vi "get_instances.vi"(6 "id (unnamed)":string, 8 "error in (no error)":errorcluster, 10 "Base Class (LabVIEW Object)":refnum<class>, 11 "Mapped Lookup in":refnum<class "Mapped Lookup.lvclass">) -> (0 "error out":errorcluster, 2 "instances":set{refnum<data-value>}(c389), 3 "Mapped Lookup out":refnum<class "Mapped Lookup.lvclass">)   [LabVIEW 2019, in "LVCOOOP.lvlib" / "Lookup API.lvlib" / "Mapped Lookup.lvclass"]
uses:
  Mapped Lookup.lvclass
  Mapped Lookup.lvclass/Mapped Lookup.ctl
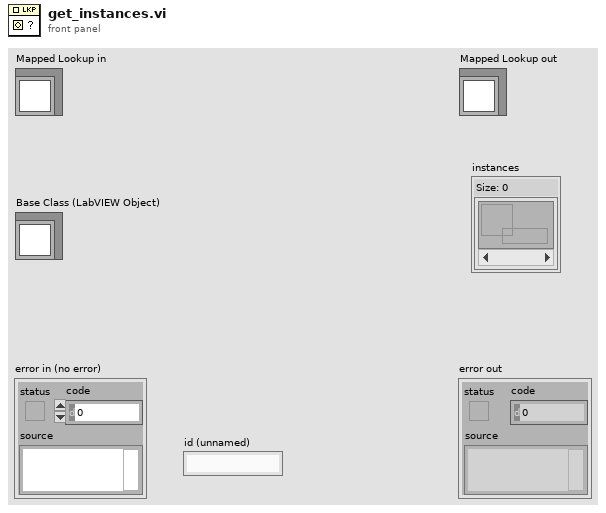
[diagram p1: front panel]
types:
  T1 = map{string, cluster{"instances":refnum<data-value>, "events":refnum<data-value>}}
  T2 = cluster{"instances":refnum<data-value>, "events":refnum<data-value>}
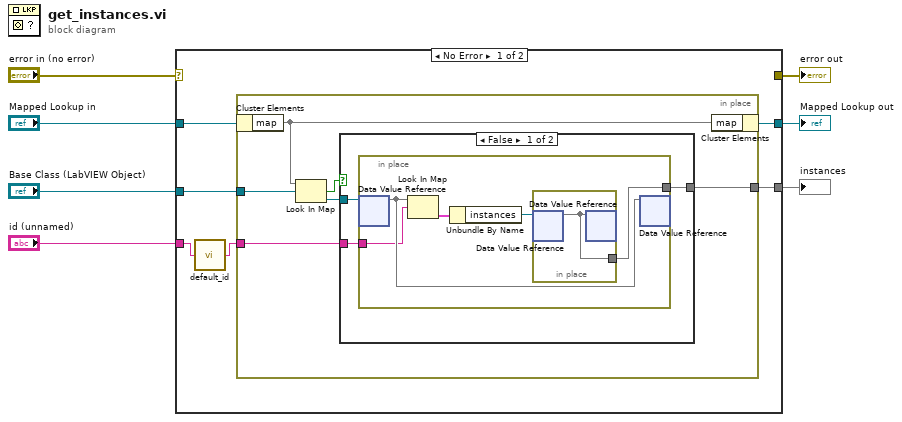
[diagram p0: block diagram]
diagram:
  n1 = case shown="No Error" "error in (no error)" {
    selector: "error in (no error)" -> [_ w30]
    tunnel: [_ w30] -> w6
    tunnel: [w10 w29] -> w5
    tunnel: "Mapped Lookup in" -> [w12 w29]
    tunnel: "id (unnamed)" -> [w13 _]
    tunnel: "Base Class (LabVIEW Object)" -> [w11 _]
    tunnel: [w8 _] -> w1
    frame No Error {
      n2 = call "default_id.vi"("id (unnamed)"=w13) -> ("String"=w9:string)
      n3 = in-place {
        in-place-border: w11 -> [w19]
        in-place-border: w9 -> [w15]
        in-place-border: [w14] -> w8
        n4 = in-place-cluster #1(w12) -> ("map"=w17:map{refnum<class>, refnum<data-value>})
        n5 = Look In Map(map=w17, key=w19) -> (key not found?=w18:bool, value=w16:refnum<data-value>)  [unwired: 1 in]
        n6 = case shown="False" w18 {
          tunnel: w16 -> [w22 _]
          tunnel: w15 -> [w21 _]
          tunnel: [w20 _] -> w14
          frame False {
            n7 = in-place {
              in-place-border: w21 -> [w26]
              in-place-border: [w23] -> w20
              n8 = in-place-dvr #2(w22) -> (w27:T1)  [unwired: 1 out]
              n9 = Look In Map(map=w27, key=w26) -> (value=w25:T2)  [unwired: 1 in, 1 out]
              n10 = Unbundle By Name(w25) -> ("instances"=w24:refnum<data-value>)
              n11 = in-place {
                in-place-border: [w28] -> w23
                n12 = in-place-dvr #3(w24) -> (w28:set{refnum<data-value>})  [unwired: 1 out]
                n13 = in-place-dvr #3(w28) -> ()  [unwired: 2 out]
              }
              n14 = in-place-dvr #2(w27) -> ()  [unwired: 2 out]
            }
          }
          frame True {
          }
        }
        n15 = in-place-cluster #1("map"=w17) -> (w10:refnum<class "Mapped Lookup.lvclass">)
      }
    }
    frame Error {
    }
  }
  "error out" <- w6
  "Mapped Lookup out" <- w5
  "instances" <- w1
